vi "Error-Get Error From List.vi"(11 "error IO":errorcluster) -> (4 "Description":string, 6 "Details":string, 10 "Found?":bool, 15 "error out":errorcluster)   [LabVIEW 2020]
uses:
  <vilib>/Utility/error.llb/DialogType.ctl
  <vilib>/Utility/config.llb/Read Key (String).vi
  <vilib>/Utility/config.llb/NI_LVConfig.lvlib
  <vilib>/regexp/Match Regular Expression.xnode
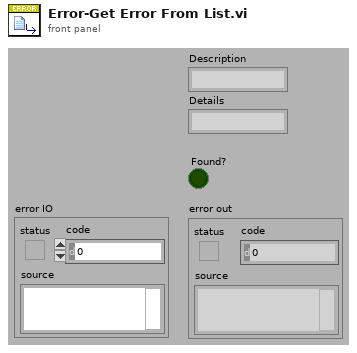
[diagram p1: front panel]
types:
  T1 = typedef "NI_LVConfig.lvlib/Config Data RefNum.ctl" = refnum<k1>
  T2 = typedef "DialogType.ctl" = u16
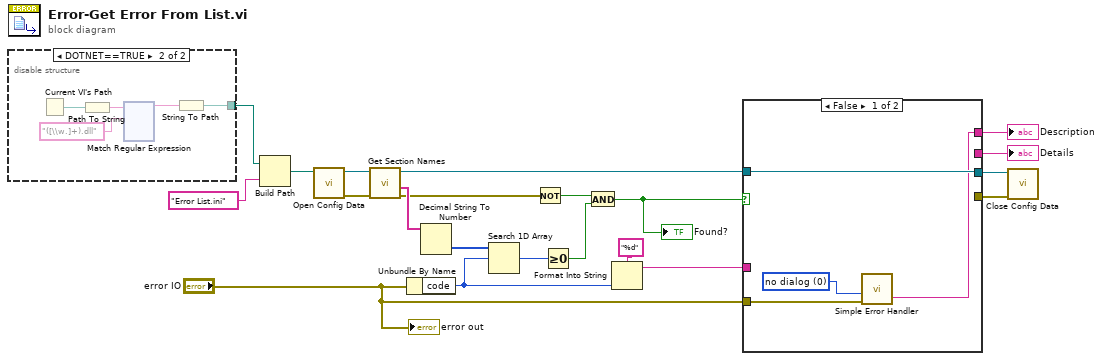
[diagram p0: block diagram]
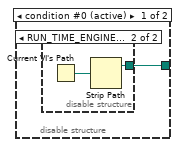
[diagram p2: hidden frame]
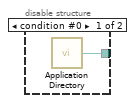
[diagram p3: hidden frame]
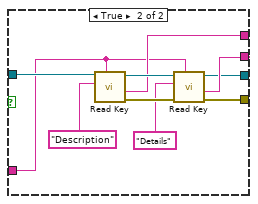
[diagram p4: hidden frame]
diagram:
  n1 = disable-structure shown="DOTNET==TRUE" {
    disable-tunnel: [w22 w26] -> w3
    frame condition #0 (active) {
      n2 = disable-structure shown="RUN_TIME_ENGINE==False, Default" {
        disable-tunnel: [w23 w24] -> w22
        frame condition #0 {
          n3 = call <vilib>:"Application Directory.vi"() -> ("Application Directory"=w23:path)
        }
        frame condition #1 (active) {
          n4 = Current VI's Path() -> (path=w25:path)
          n5 = Strip Path(path=w25) -> (stripped path=w24:path)  [unwired: 1 out]
        }
      }
    }
    frame condition #1 {
      n6 = Current VI's Path() -> (path=w30:path)
      n7 = Path To String(path=w30) -> (string=w29:string)
      n8 = xnode "Match Regular Expression"("input string"=w29, "regular expression"="([\\w.]+).dll") -> ("before match"=w27:string)  [unwired: 4 in, 4 out]
      n9 = String To Path(string=w27) -> (path=w26:path)
    }
  }
  n10 = Build Path(base path=w3, name or relative path="Error List.ini") -> (appended path=w1:path)
  n11 = call <vilib>:"Open Config Data.vi"("configuration file path"=w1) -> ("error out"=w18:errorcluster, "refnum"=w17:T1)  [unwired: 8 in, 1 out]
  n12 = call <vilib>:"Get Section Names.vi"("error in (no error)"=w18, "refnum"=w17) -> ("error out"=w12:errorcluster, "section names"=w19:string[], "refnum out"=w13:T1)  [unwired: 7 in]
  n13 = Unbundle By Name("error IO") -> ("code"=w10:i32)
  n14 = Decimal String To Number(string=w19) -> (number=w20:i32[])  [unwired: 2 in, 1 out]
  n15 = Search 1D Array(1D array=w20, element=w10) -> (index of element=w21:i32)  [unwired: 1 in]
  n16 = Not(x=w12) -> (.not. x?=w15:bool)
  n17 = Greater Or Equal To 0?(x=w21) -> (x >= 0?=w14:bool)
  n18 = And(x=w15, y=w14) -> (x .and. y?=w4:bool)
  "Found?" <- w4
  n19 = Format Into String(format string="%d", w10) -> (resulting string=w9:string)  [unwired: 2 in, 1 out]
  n20 = case shown="False" w4 {
    tunnel: w13 -> [w148 w158]
    tunnel: w9 -> [_ w149]
    tunnel: [w146 w153] -> w6
    tunnel: [_ w152] -> w5
    tunnel: [w148 w150] -> w8
    tunnel: [_ w151] -> w7
    tunnel: "error IO" -> [w147 _]
    frame False {
      w145 = T2 0 items=["no dialog", "OK message", "continue or stop message", "OK message + warnings", "continue/stop + warnings"] ("type of dialog (OK msg:1)")
      n21 = call <vilib>:"Simple Error Handler.vi"("type of dialog (OK msg:1)"=w145, "error in (no error)"=w147) -> ("message"=w146:string)  [unwired: 3 in, 4 out]
    }
    frame True {
      n22 = call-poly <vilib>:"Read Key.vi"("section"=w149, "key"="Description", "refnum"=w158) -> ("error out"=w155:errorcluster, "value"=w153:string, "refnum out"=w156:T1)  [unwired: 5 in, 1 out]
      n23 = call-poly <vilib>:"Read Key.vi"("section"=w149, "error in (no error)"=w155, "key"="Details", "refnum"=w156) -> ("error out"=w151:errorcluster, "value"=w152:string, "refnum out"=w150:T1)  [unwired: 4 in, 1 out]
    }
  }
  "Description" <- w6
  "Details" <- w5
  n24 = call <vilib>:"Close Config Data.vi"("error in (no error)"=w7, "refnum"=w8) -> ()  [unwired: 8 in, 2 out]
  "error out" <- "error IO"
